vi "Init IL Action.vi"(5 "Message Priority (Normal)":T1=enum."Normal", 6 "IL Action (Stop if Default)":refnum<class "Message.lvclass">, 7 "Destination Enqueuer (Default)":refnum<class "Message Enqueuer.lvclass">, 8 "error in (no error)":errorcluster, 11 "IL Action in":refnum<class "IL Action.lvclass">) -> (0 "error out":errorcluster, 3 "IL Action out":refnum<class "IL Action.lvclass">)   [LabVIEW 2015, in "Interlocks.lvlib" / "IL Action.lvclass"]
uses:
  IL Action.lvclass
  <vilib>/ActorFramework/Message/Message.lvclass
  <vilib>/ActorFramework/Message Enqueuer/Message Enqueuer.lvclass
  <vilib>/ActorFramework/Message Enqueuer/Message Priority.ctl
  <vilib>/ActorFramework/Stop Msg/Stop Msg.lvclass
  IL Action.lvclass/IL Action.ctl
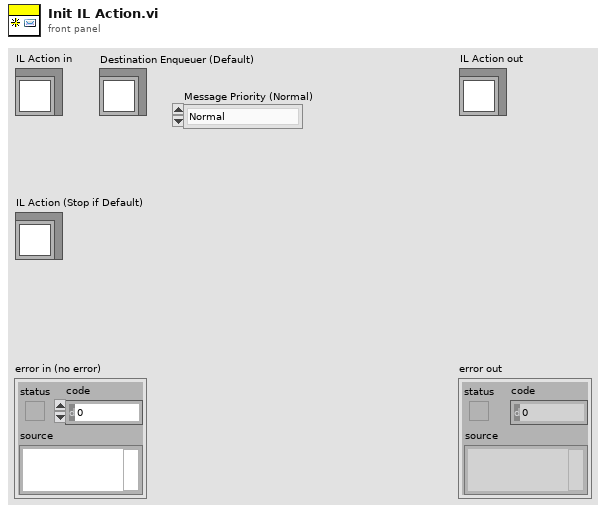
[diagram p1: front panel]
types:
  T1 = typedef "Actor Framework.lvlib/Message Enqueuer.lvclass/Message Priority.ctl" = enum16{"Low", "Normal", "High"}
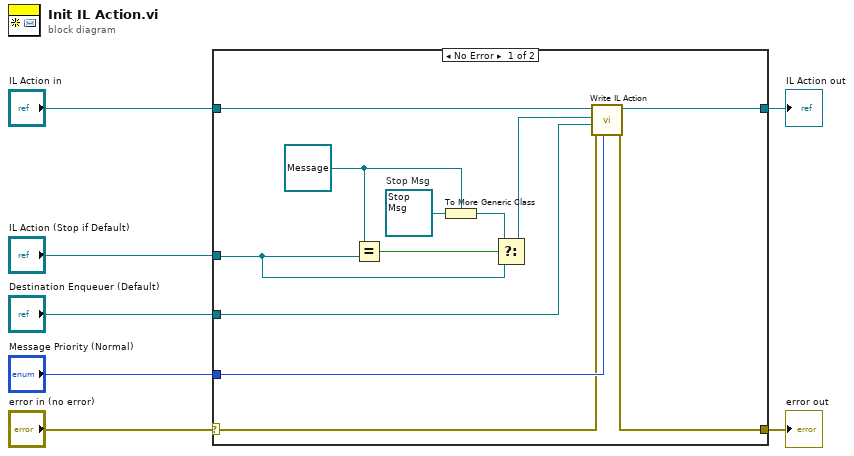
[diagram p0: block diagram]
diagram:
  n1 = case shown="No Error" "error in (no error)" {
    selector: "error in (no error)" -> [w9 w21]
    tunnel: [w8 w21] -> w6
    tunnel: [w18 w20] -> w4
    tunnel: "IL Action in" -> [w19 w20]
    tunnel: "IL Action (Stop if Default)" -> [w16 _]
    tunnel: "Destination Enqueuer (Default)" -> [w11 _]
    tunnel: "Message Priority (Normal)" -> [w10 _]
    frame No Error {
      w15 = refnum<class "Stop Msg.lvclass"> refnum  # Stop Msg
      w13 = refnum<class "Message.lvclass"> refnum ("IL Action (Stop if Default)")
      n2 = Equal?(x=w13, y=w16) -> (x = y?=w17:bool)
      n3 = To More Generic Class(target class=w13, reference=w15) -> (generic class reference=w14:refnum<class "Message.lvclass">)
      n4 = Select(t=w14, s=w17, f=w16) -> (s? t:f=w12:refnum<class "Message.lvclass">)
      n5 = call "Write IL Action.vi"("Message Priority"=w10, "error in (no error)"=w9, "Destination Enqueuer"=w11, "Actor Framework:Message"=w12, "IL Action in"=w19) -> ("error out"=w8:errorcluster, "IL Action out"=w18:refnum<class "IL Action.lvclass">)  [unwired: 5 in]
    }
    frame Error {
    }
  }
  "error out" <- w6
  "IL Action out" <- w4
